vi "Feeding.vi"(8 "error In":errorcluster) -> (0 "error out":errorcluster)   [LabVIEW 2017]
uses:
  <vilib>/Utility/error.llb/DialogType.ctl
  Controls/Feed_Cyc_Data.ctl
  Controls/QUEUE_STATES.ctl
  Controls/Feed_St.ctl
  <vilib>/Utility/file.llb/Read Delimited Spreadsheet (string).vi
  Global/PLC_to_Auto.vi
  <vilib>/Instr/_visa.llb/VISA Configure Serial Port (Instr).vi
panel:
  in  "Door Number 2":i32
  out "Door Number":i32
  out "Door":bool
  out "number":i32
  out "Scanned Chld Part.Selected Door No":string
  out "output cluster":cluster{"Feeder Door Open":bool, "Address":u16}
  out "Scanned Chld Part":T1
  in  "Close _Door":bool
  out "raw scan code":string
  in  "Boolean":bool
  in  "String":string
  out "Bins/Box":i32
  out "Scanner Comm":bool
  out "Stop scanner":bool
  out "CYCLE STATUS":string
  out "CURRENT PLAN":T2
  out "SCAN CODE:":string
  out "Selected Plan structure":string[][](table)
  out "Plan Selected:":string
  out "USER:-":string
  in  "Stop":bool
  out "DATE/TIME":string
  out "Screen Name":string
  # "DOOR NUMBER"
  # "FEEDER STATUS"
  # "DOOR NUMBER"
  # "FEEDER STATUS"
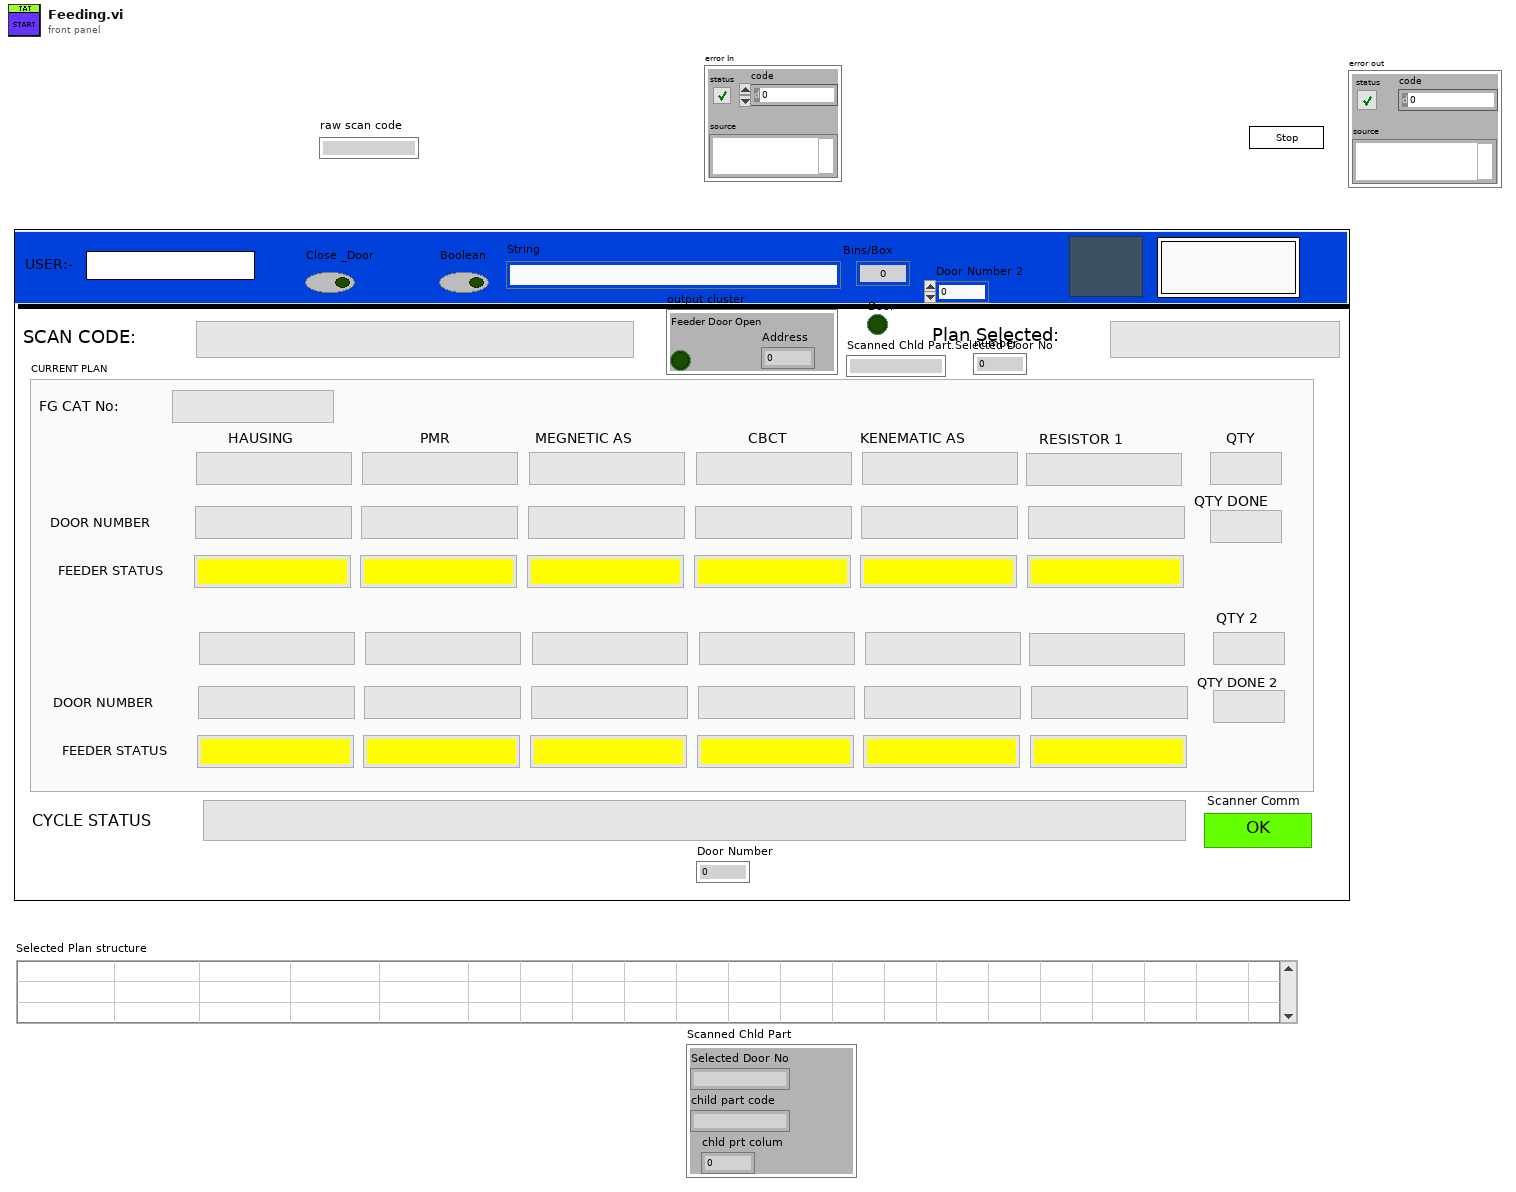
[diagram p1: front panel]
types:
  T1 = cluster{"Selected Door No":string, "child part code":string, "chld prt colum":i32}
  T2 = cluster{"FG CAT No:":string, "HAUSING":string, "PMR":string, "MEGNETIC AS":string, "CBCT":string, "KENEMATIC AS":string, "RESISTOR 1":string, "HAUSING DOOR":string, "PMR DOOR":string, "MAGNETIC AS DOOR":string, "CBCT DOOR":string, "KINEMATIC AS DOOR":string, "RESISTOR 1 DOOR":string, "HAUSING FEED STATUS":string, "PMR FEED STATUS":string, "MAGNETIC AS FEEED STATUS":string, "CBCT FEED STATUS":string, "KINEMATIC AS FEED STATUS":string, "RESISTOR 1 FEED STATUS":string, "QTY":string, "QTY DONE":string, "HAUSING 2":string, "PMR 2":string, "MEGNETIC AS 2":string, "CBCT 2":string, "KENEMATIC AS 2":string, "RESISTOR 2":string, "HAUSING DOOR 2":string, "PMR DOOR 2":string, "MAGNETIC AS DOOR 2":string, "CBCT DOOR 2":string, "KINEMATIC AS DOOR 2":string, "RESISTOR 1 DOOR 2":string, "HAUSING FEED STATUS 2":string, "PMR FEED STATUS 2":string, "MAGNETIC AS FEEED STATUS 2":string, "CBCT FEED STATUS 2":string, "KINEMATIC AS FEED STATUS 2":string, "RESISTOR 1 FEED STATUS 2":string, "QTY 2":string, "QTY DONE 2":string}
  T3 = typedef "Feed_Cyc_Data.ctl" = cluster{"Cycle_Plan":path, "Plan_Data":string[][], "Scanned_Data":string[], "Scanned Chld Part":cluster{"Selected Door No":string, "child part code":string, "chld prt Row":i32, "Chld Prt Index":i32, "Scanned Data":string}, "feed Status Indi":refnum<vi>[], "Recipe Selected":cluster{"Bin/Box Mode":i32, "Selected Section":i32}}
  T4 = typedef "DialogType.ctl" = u16
  T5 = enum32{"invalid app kind", "Development System", "Run Time System", "Student Edition", "Embedded LabVIEW", "Evaluation", "Custom"}
  T6 = typedef "QUEUE_STATES.ctl" = enum16{"CREATE Q", "EN Q", "DE Q", "CLOSE Q"}
  T7 = cluster{"Printer IP":string, "PLC IP Address":string, "Scanner Com":refnum<visa-resource-name>}
  T8 = typedef "Feed_St.ctl" = enum16{"Package_Qty_Count", "GENERATE_QR_PRNT", "Cluster_update", "Read_Plan", "QR_Scanned", "Int", "SaveReport ", "Open_Door", "Error_Handler", "Wait", "Close_Door", "Stop"}
  T9 = cluster{"Selected Door No":string, "child part code":string, "chld prt Row":i32, "Chld Prt Index":i32, "Scanned Data":string}
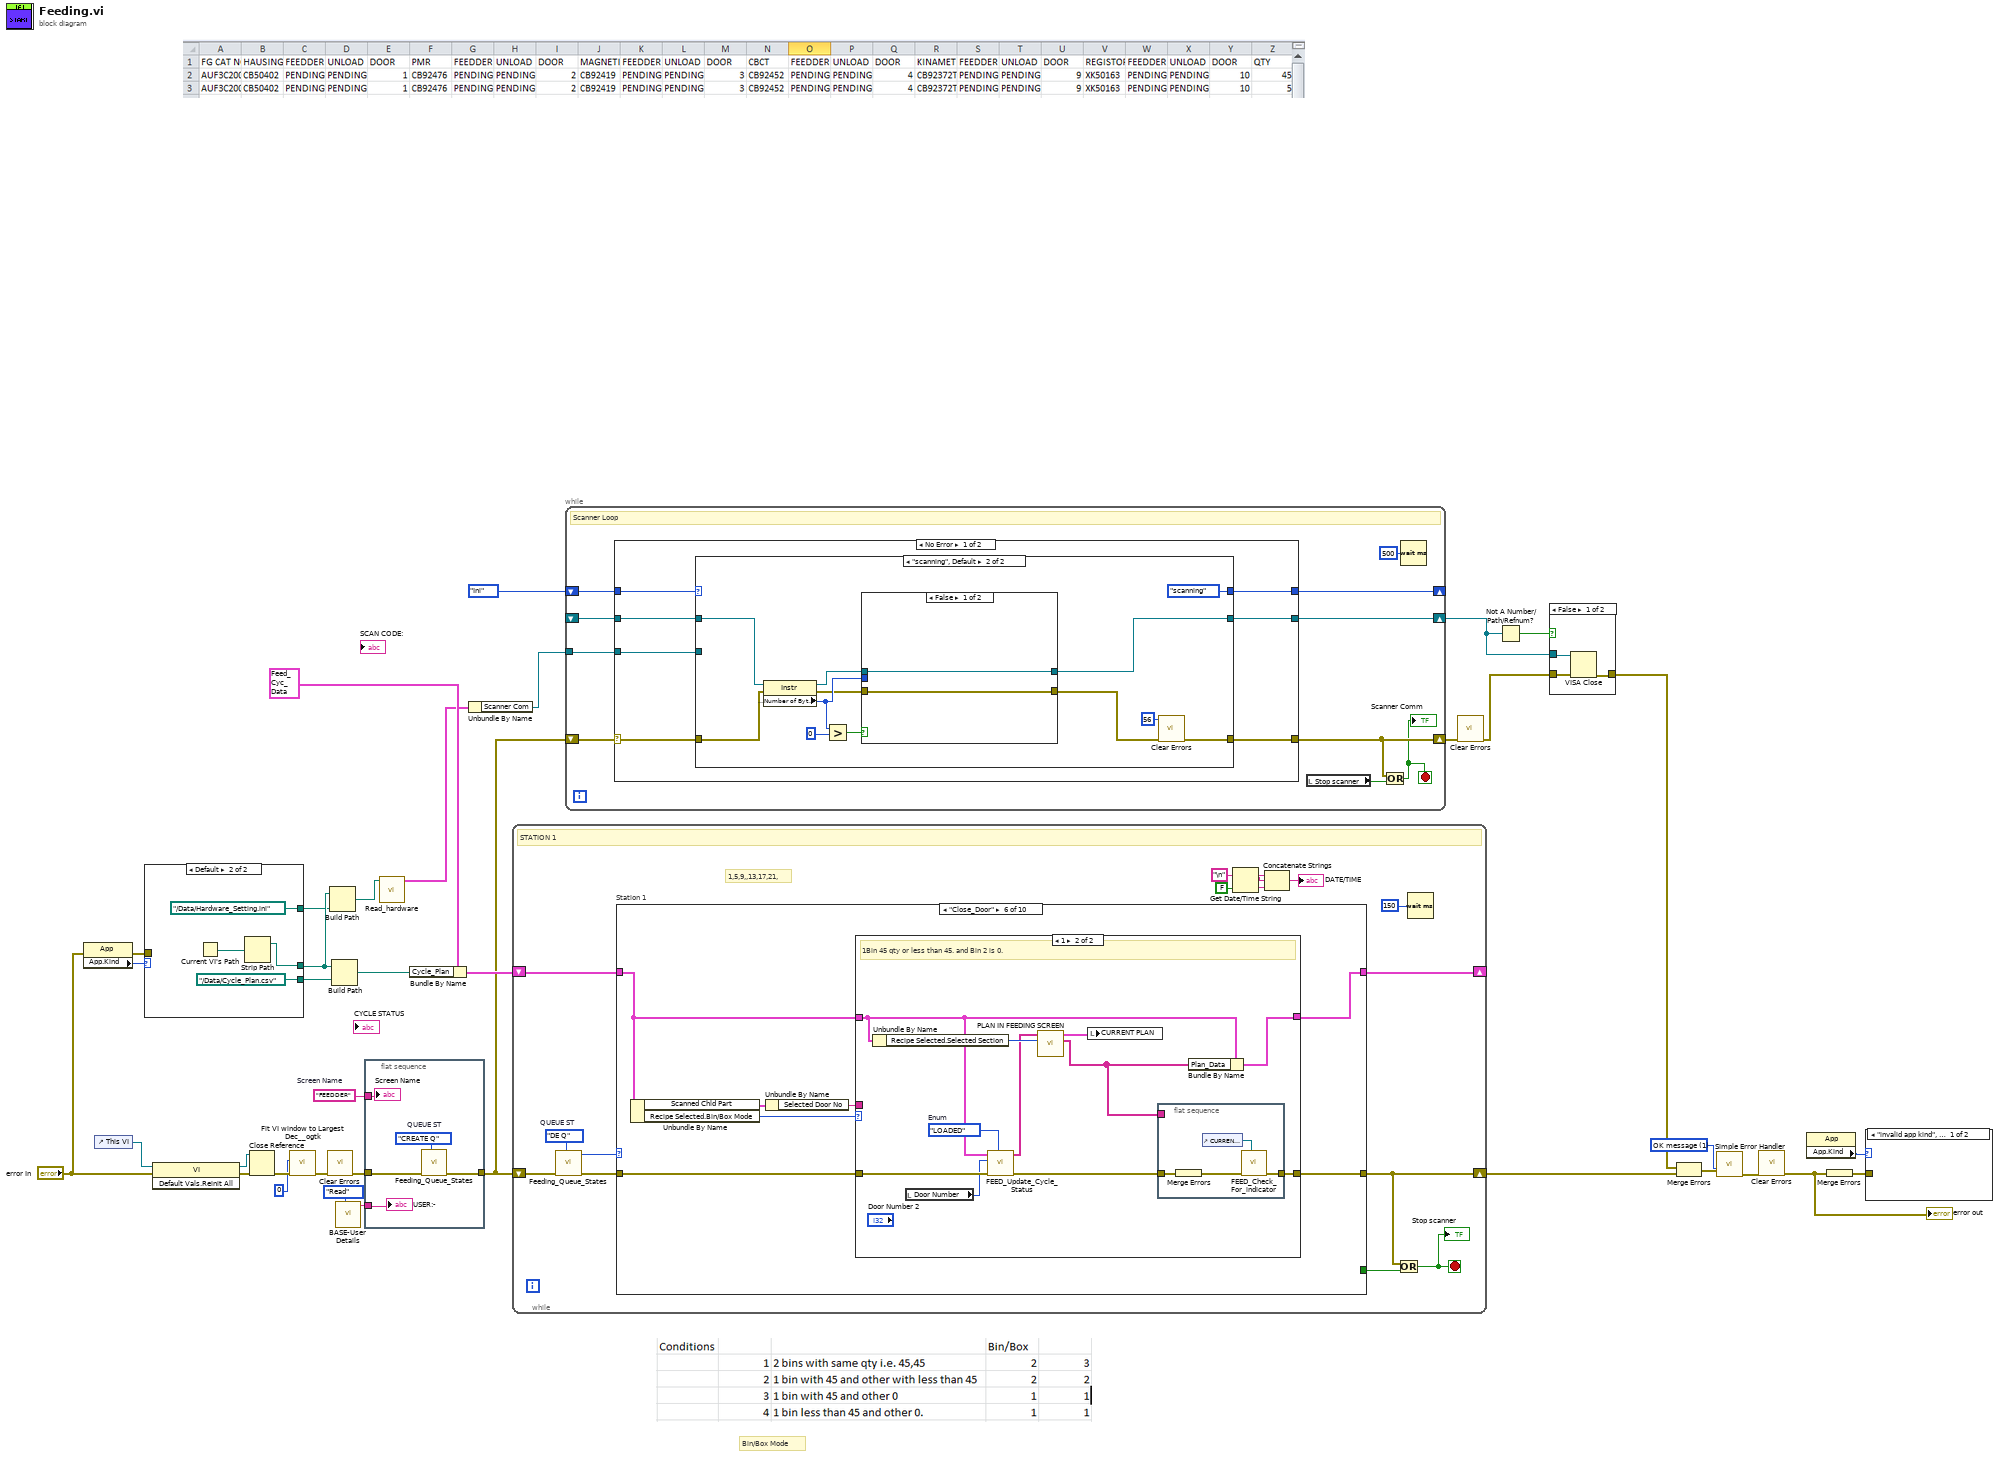
[diagram p0: block diagram]
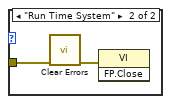
[diagram p2: hidden frame]
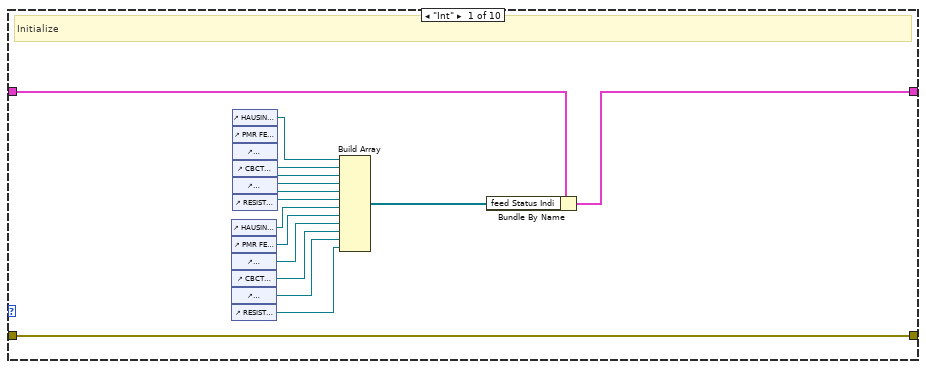
[diagram p3: hidden frame]
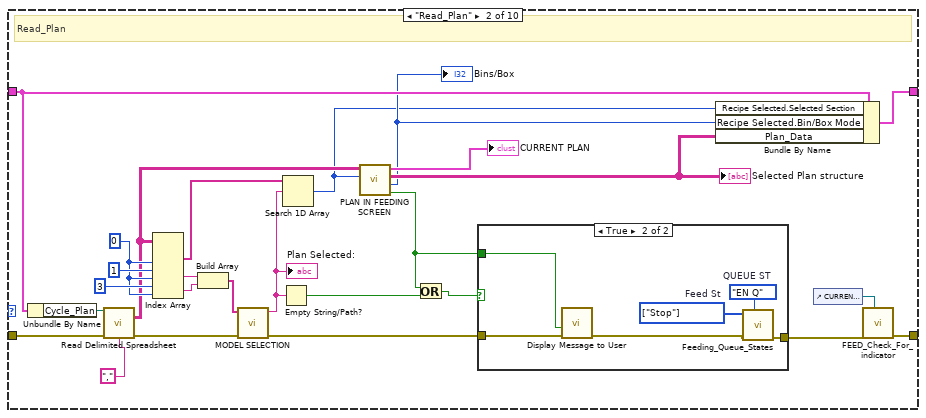
[diagram p4: hidden frame]
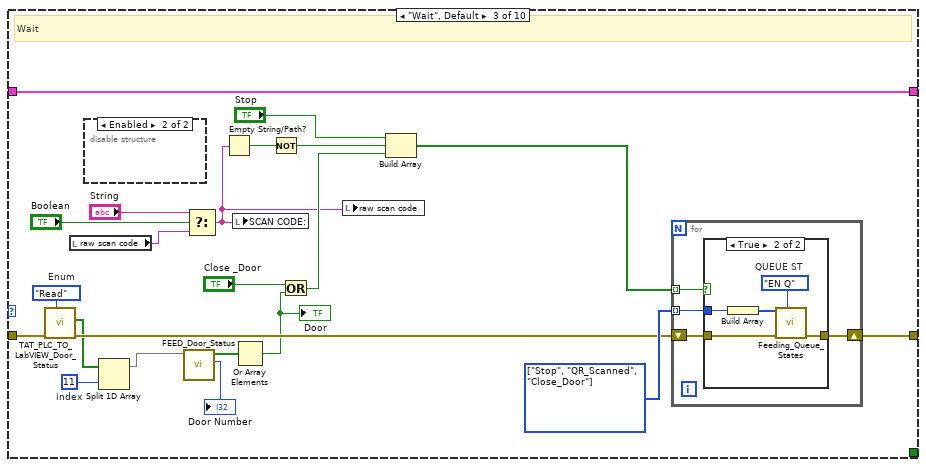
[diagram p6: hidden frame]
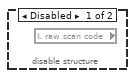
[diagram p7: hidden frame]
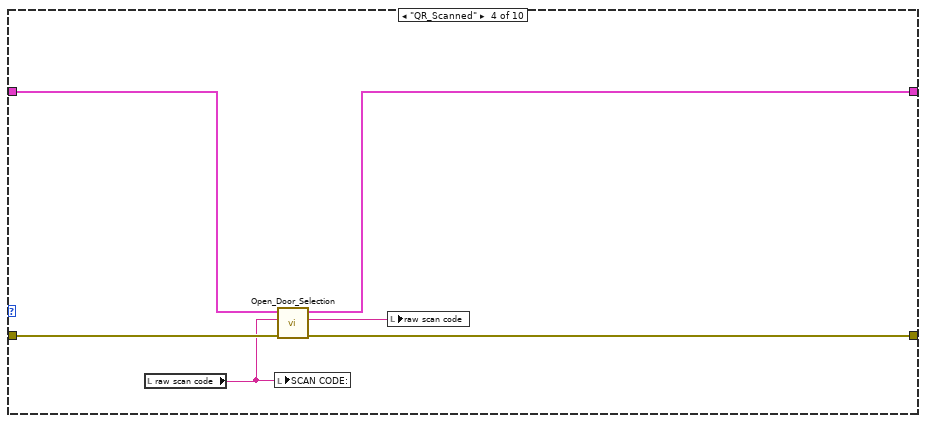
[diagram p9: hidden frame]
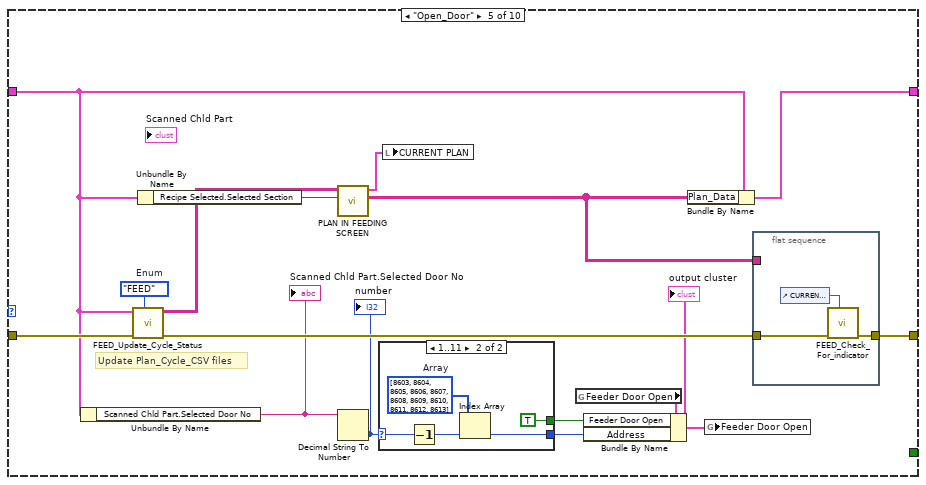
[diagram p10: hidden frame]
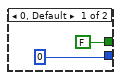
[diagram p11: hidden frame]
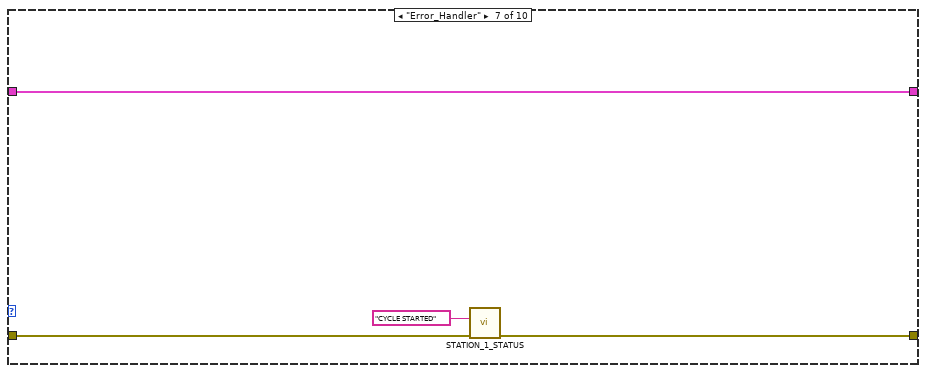
[diagram p13: hidden frame]
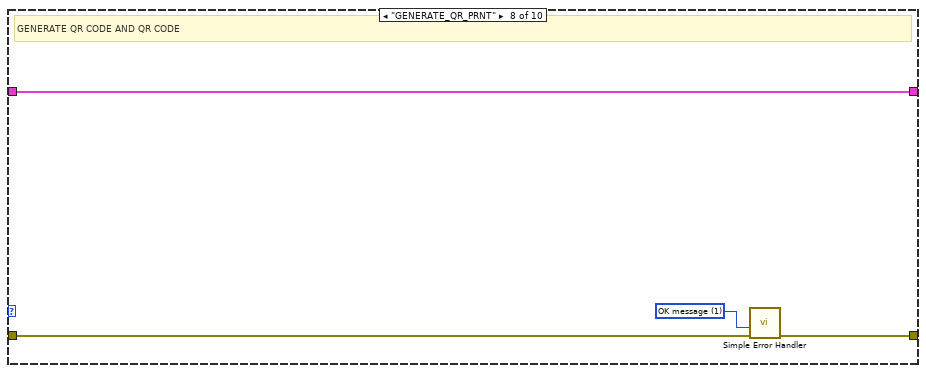
[diagram p14: hidden frame]
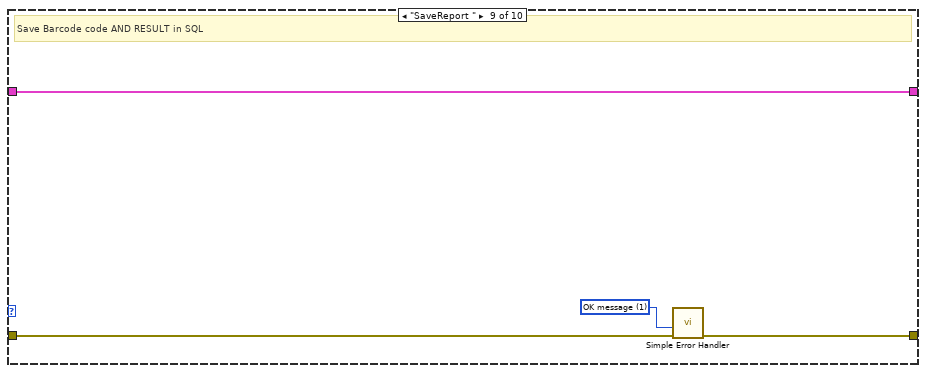
[diagram p15: hidden frame]
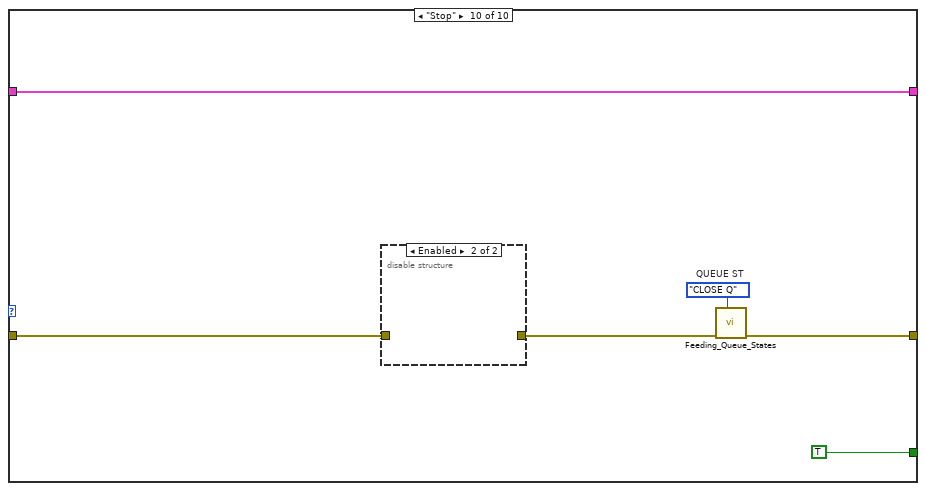
[diagram p16: hidden frame]
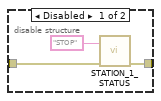
[diagram p17: hidden frame]
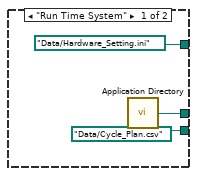
[diagram p18: hidden frame]
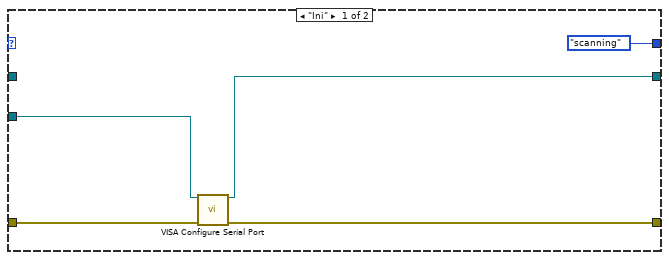
[diagram p20: hidden frame]
diagram:
  w17 = "FEEDDER"  # Screen Name
  w29 = T4 1 items=["no dialog", "OK message", "continue or stop message", "OK message + warnings", "continue/stop + warnings"] ("type of dialog (OK msg:1)")
  # "Bin/Box Mode"
  n1 = property class="App"(error in="error In") -> (error out=w25:errorcluster, "App.Kind"=w27:T5)  [unwired: 1 in, 1 out]
  n2 = control-ref of="This VI"() -> (w36:refnum<vi>)
  n3 = case shown="Default" w27 {
    tunnel: [path "Data/Cycle_Plan.csv" ("path") path "../Data/Cycle_Plan.csv" ("path")] -> w26
    tunnel: [w37 w41] -> w6
    tunnel: w25 -> [_ _]
    tunnel: [path "Data/Hardware_Setting.ini" ("path") path "../Data/Hardware_Setting.ini" ("path")] -> w5
    frame "Run Time System" {
      n4 = call <vilib>:"Application Directory.vi"() -> ("Application Directory"=w37:path)
    }
    frame Default {
      n5 = Current VI's Path() -> (path=w42:path)
      n6 = Strip Path(path=w42) -> (stripped path=w41:path)  [unwired: 1 out]
    }
  }
  n7 = invoke class="VI" method="Default Vals.Reinit All"(reference=w36, error in="error In") -> (reference out=w34:refnum<vi>, error out=w35:errorcluster)  [unwired: 1 in, 1 out]
  n8 = Close Reference(reference=w34, error in (no error)=w35) -> (error out=w33:errorcluster)
  n9 = call <userlib>:"Fit VI window to Largest Dec__ogtk.vi"("error in (no error)"=w33, "border spacing (2 px)"=0) -> ("error out"=w23:errorcluster)  [unwired: 4 in, 1 out]
  n10 = call <vilib>:"Clear Errors.vi"("error in (no error)"=w23) -> ("error out"=w10:errorcluster)  [unwired: 5 in, 1 out]
  n11 = Build Path(base path=w6, name or relative path=w5) -> (appended path=w4:path)
  n12 = Build Path(base path=w6, name or relative path=w26) -> (appended path=w19:path)
  n13 = call "BASE-User Details.vi"("Enum"=enum16{"Read", "Write"}."Read") -> ("User Name Out"=w30:string)  [unwired: 9 in, 1 out]
  n14 = flat-sequence {
    tunnel: [w45] -> w11
    tunnel: w10 -> [w46]
    tunnel: w30 -> [w48]
    tunnel: w17 -> [w47]
    frame #0 {
      w44 = QUEUE_STATES."CREATE Q"  # QUEUE ST
      n15 = call "Feeding_Queue_States.vi"("QUEUE ST"=w44, "error in"=w46) -> ("error OUT"=w45:errorcluster)  [unwired: 8 in, 1 out]
      "USER:-" <- w48
      "Screen Name" <- w47
    }
  }
  n16 = call "Read_hardware.vi"("configuration file path"=w4) -> ("data"=w8:T7)  [unwired: 10 in]
  n17 = Bundle By Name(cluster=T3 {"Cycle_Plan"=path "", "Plan_Data"=[], "Scanned_Data"=[], "Scanned Chld Part"={"Selected Door No"="", "child part code"="", "chld prt Row"=0, "Chld Prt Index"=0, "Scanned Data"=""}, "feed Status Indi"=[], "Recipe Selected"={"Bin/Box Mode"=0, "Selected Section"=0}}, "Cycle_Plan"=w19) -> (w18:T3)
  n18 = Unbundle By Name(w8) -> ("Scanner Com"=w7:refnum<visa-resource-name>)
  n19 = while {
    shift-right: [w55] -> _
    shift-left: w18 -> [w56]
    shift-right: [w53] -> w9
    shift-left: w11 -> [w52]
    stop <- w54 stop-if-true
    w50 = QUEUE_STATES."DE Q"  # QUEUE ST
    # "1,5,9,,13,17,21,"
    # "STATION 1"
    n20 = call "Feeding_Queue_States.vi"("QUEUE ST"=w50, "error in"=w52) -> ("error OUT"=w51:errorcluster, "Feed ST"=w49:T8)  [unwired: 8 in]
    n21 = case "Station 1" shown="\"Close_Door\"" w49 {
      tunnel: [_ _ _ _ _ _ _ _ _ TRUE] -> w57
      tunnel: [w79 w85 w131 w149 w164 w182 w202 w207 w211 w213] -> w53
      tunnel: w51 -> [w79 w104 w121 w150 w166 w183 w203 w206 w210 w217]
      tunnel: w56 -> [w66 w94 w134 w147 w157 w179 w201 w205 w209 w216]
      tunnel: [w65 w84 w134 w146 w161 w178 w201 w205 w209 w216] -> w55
      frame "Int" {
        # "Initialize"
        n22 = control-ref of="HAUSING FEED STATUS 2"() -> (w73:refnum<vi>)
        n23 = control-ref of="PMR FEED STATUS 2"() -> (w74:refnum<vi>)
        n24 = control-ref of="MAGNETIC AS FEEED STATUS 2"() -> (w75:refnum<vi>)
        n25 = control-ref of="CBCT FEED STATUS 2"() -> (w76:refnum<vi>)
        n26 = control-ref of="KINEMATIC AS FEED STATUS 2"() -> (w77:refnum<vi>)
        n27 = control-ref of="RESISTOR 1 FEED STATUS 2"() -> (w78:refnum<vi>)
        n28 = control-ref of="HAUSING FEED STATUS"() -> (w67:refnum<vi>)
        n29 = control-ref of="PMR FEED STATUS"() -> (w68:refnum<vi>)
        n30 = control-ref of="MAGNETIC AS FEEED STATUS"() -> (w69:refnum<vi>)
        n31 = control-ref of="CBCT FEED STATUS"() -> (w70:refnum<vi>)
        n32 = control-ref of="KINEMATIC AS FEED STATUS"() -> (w71:refnum<vi>)
        n33 = control-ref of="RESISTOR 1 FEED STATUS"() -> (w72:refnum<vi>)
        n34 = Build Array(w67, w68, w69, w70, w71, w72, w73, w74, w75, w76, w77, w78) -> (w64:refnum<vi>[])
        n35 = Bundle By Name(cluster=w66, "feed Status Indi"=w64) -> (w65:T3)
      }
      frame "Read_Plan" {
        w96 = 0
        # "Read_Plan"
        n36 = Unbundle By Name(w94) -> ("Cycle_Plan"=w103:path)
        n37 = call-poly <vilib>:"Read Delimited Spreadsheet.vi"("file path (dialog if empty)"=w103, "error in (no error)"=w104, "delimiter (\\t)"=",") -> ("all rows"=w90:string[][], "error out"=w97:errorcluster)  [unwired: 7 in, 4 out]
        n38 = Index Array(array=w90, index (col) #1=w96, index (row) #2=1, index (col) #2=w96, index (row) #3=3, index (col) #3=w96) -> (element #1=w95:string[], element #2=w100:string, element #3=w99:string)  [unwired: 1 in]
        n39 = Build Array(w100, w99) -> (w98:string[])
        n40 = call "MODEL SELECTION.vi"("error in (no error)"=w97, "Plan List"=w98) -> ("error out 2"=w88:errorcluster, "Plan Selected"=w93:string)  [unwired: 8 in]
        "Plan Selected:" <- w93
        n41 = Empty String/Path?(string/path=w93) -> (empty?=w87:bool)
        n42 = Search 1D Array(1D array=w95, element=w93) -> (index of element=w82:i32)  [unwired: 1 in]
        n43 = call "PLAN IN FEEDING SCREEN.vi"("Section selected"=w82, "PLAN In"=w90) -> ("FEED CMPLT?"=w80:bool, "Bin/Box"=w89:i32, "PLAN Out"=w91:string[][], "CURRENT PLAN"=→"CURRENT PLAN":T2)  [unwired: 6 in]
        "Selected Plan structure" <- w91
        "Bins/Box" <- w89
        n44 = Or(x=w80, y=w87) -> (x .or. y?=w81:bool)
        n45 = case shown="True" w81 {
          tunnel: w88 -> [w106 w109]
          tunnel: [w106 w111] -> w86
          tunnel: w80 -> [_ w107]
          frame False {
          }
          frame True {
            w110 = T8[] [enum."Stop"] items=["Package_Qty_Count", "GENERATE_QR_PRNT", "Cluster_update", "Read_Plan", "QR_Scanned", "Int", "SaveReport ", "Open_Door", "Error_Handler", "Wait", "Close_Door", "Stop"]  # Feed St
            w112 = QUEUE_STATES."EN Q"  # QUEUE ST
            n46 = call "Display Message to User"("error in (no error)"=w109, "Enable"=w107) -> ("error out"=w108:errorcluster)  [unwired: 8 in, 1 out]
            n47 = call "Feeding_Queue_States.vi"("QUEUE ST"=w112, "error in"=w108, "Feed St"=w110) -> ("error OUT"=w111:errorcluster)  [unwired: 7 in, 1 out]
          }
        }
        n48 = Bundle By Name(cluster=w94, "Recipe Selected.Selected Section"=w82, "Recipe Selected.Bin/Box Mode"=w89, "Plan_Data"=w91) -> (w84:T3)
        n49 = control-ref of="CURRENT PLAN"() -> (w83:refnum<vi>)
        n50 = call "FEED_Check_For_indicator.vi"("CURRENT PLAN"=w83, "error in (no error)"=w86) -> ("error out"=w85:errorcluster)  [unwired: 9 in]
      }
      frame "Wait", Default {
        w113 = 11  # index
        w124 = enum16{"Read", "Write"}."Read"  # Enum
        w127 = T8[] [enum."Stop", enum."QR_Scanned", enum."Close_Door"] items=["Package_Qty_Count", "GENERATE_QR_PRNT", "Cluster_update", "Read_Plan", "QR_Scanned", "Int", "SaveReport ", "Open_Door", "Error_Handler", "Wait", "Close_Door", "Stop"] ("Array")
        # "Wait"
        n51 = call "TAT_PLC_TO_LabVIEW_Door_Status.vi"("Enum"=w124, "error in (no error)"=w121) -> ("error out"=w120:errorcluster, "Array 2"=w115:bool[])  [unwired: 8 in]
        n52 = local read "raw scan code"() -> (w125:string)
        n53 = disable-structure shown="Enabled" {
          frame Disabled {
            n54 = local read "raw scan code"() -> ()  [unwired: 1 out]
          }
          frame Enabled {
          }
        }
        n55 = Split 1D Array(array=w115, index=w113) -> (first subarray=w114:bool[])  [unwired: 1 out]
        n56 = call "FEED_Door_Status.vi"("Array in"=w114) -> ("Door Number"=→"Door Number":i32, "Array out"=w119:bool[])  [unwired: 9 in]
        n57 = Select(t="String", s="Boolean", f=w125) -> (s? t:f=w116:string)
        n58 = Empty String/Path?(string/path=w116) -> (empty?=w130:bool)
        n59 = local write "SCAN CODE:"(w116) -> ()
        n60 = Or Array Elements(Boolean array=w119) -> (logical OR=w118:bool)
        "Door" <- w118
        n61 = Not(x=w130) -> (.not. x?=w126:bool)
        n62 = Or(x="Close _Door", y=w118) -> (x .or. y?=w122:bool)
        n63 = local write "raw scan code"(w116) -> ()
        n64 = Build Array("Stop", w126, w122) -> (w128:bool[])
        n65 = for {
          shift-right: [w137] -> w131
          shift-left: w120 -> [w138]
          tunnel: w128 -> [w136] mode=indexing
          tunnel: w127 -> [w135] mode=indexing
          n66 = case shown="True" w136 {
            tunnel: w138 -> [w139 w143]
            tunnel: [w139 w142] -> w137
            tunnel: w135 -> [_ w141]
            frame False {
            }
            frame True {
              w144 = QUEUE_STATES."EN Q"  # QUEUE ST
              n67 = Build Array(w141) -> (w140:T8[])
              n68 = call "Feeding_Queue_States.vi"("QUEUE ST"=w144, "error in"=w143, "Feed St"=w140) -> ("error OUT"=w142:errorcluster)  [unwired: 7 in, 1 out]
            }
          }
        }
      }
      frame "QR_Scanned" {
        n69 = local read "raw scan code"() -> (w148:string)
        n70 = local write "SCAN CODE:"(w148) -> ()
        n71 = call "Open_Door_Selection.vi"("error in (no error)"=w150, "raw scan code"=w148, "Cluster In"=w147) -> ("error out"=w149:errorcluster, "String"=w145:string, "Cluster Out"=w146:T3)  [unwired: 6 in]
        n72 = local write "raw scan code"(w145) -> ()
      }
      frame "Open_Door" {
        w159 = enum16{"FEED", "LOADED"}."FEED"  # Enum
        # "Update Plan_Cycle_CSV files"
        n73 = Unbundle By Name(w157) -> ("Scanned Chld Part.Selected Door No"=w153:string)
        "Scanned Chld Part.Selected Door No" <- w153
        n74 = call "FEED_Update_Cycle_Status.vi"("Enum"=w159, "error in (no error)"=w166, 11:w157) -> ("error out"=w165:errorcluster, "output array"=w158:string[][])  [unwired: 6 in, 1 out]
        n75 = Unbundle By Name(w157) -> ("Recipe Selected.Selected Section"=w163:i32)
        n76 = call "PLAN IN FEEDING SCREEN.vi"("Section selected"=w163, "PLAN In"=w158) -> ("PLAN Out"=w160:string[][], "CURRENT PLAN"=w162:T2)  [unwired: 6 in, 2 out]
        n77 = Decimal String To Number(string=w153) -> (number=w154:i32)  [unwired: 2 in, 1 out]
        "number" <- w154
        n78 = case shown="1..11" w154 {
          selector: w154 -> [_ w173]
          tunnel: [u16 0 w172] -> w152
          tunnel: [FALSE TRUE] -> w151
          frame 0, Default {
          }
          frame 1..11 {
            w169 = i32[] [8603, 8604, 8605, 8606, 8607, 8608, 8609, 8610, 8611, 8612, 8613]  # Array
            n79 = Decrement(x=w173) -> (x-1=w170:i32)
            n80 = Index Array(array=w169, index=w170) -> (element=w172:i32)
          }
        }
        n81 = local write "CURRENT PLAN"(w162) -> ()
        n82 = global read "PLC_to_Auto.vi" "Feeder Door Open"() -> (w156:cluster{"Feeder Door Open":bool, "Address":u16})
        n83 = Bundle By Name(cluster=w156, "Feeder Door Open"=w151, "Address"=w152) -> (w155:cluster{"Feeder Door Open":bool, "Address":u16})
        "output cluster" <- w155
        n84 = Bundle By Name(cluster=w157, "Plan_Data"=w160) -> (w161:T3)
        n85 = global write "PLC_to_Auto.vi" "Feeder Door Open"(w155) -> ()
        n86 = flat-sequence {
          tunnel: w165 -> [w176]
          tunnel: [w175] -> w164
          tunnel: w160 -> [_]
          frame #0 {
            n87 = control-ref of="CURRENT PLAN"() -> (w174:refnum<vi>)
            n88 = call "FEED_Check_For_indicator.vi"("CURRENT PLAN"=w174, "error in (no error)"=w176) -> ("error out"=w175:errorcluster)  [unwired: 9 in]
          }
        }
      }
      frame "Close_Door" {
        n89 = Unbundle By Name(w179) -> ("Scanned Chld Part"=w180:T9, "Recipe Selected.Bin/Box Mode"=w177:i32)
        n90 = Unbundle By Name(w180) -> ("Selected Door No"=w181:string)
        n91 = case shown="1" w177 {
          tunnel: w183 -> [w184 w195]
          tunnel: [w184 w188] -> w182
          tunnel: w181 -> [_ _]
          tunnel: w179 -> [w185 w190]
          tunnel: [w185 w196] -> w178
          frame 0, Default {
          }
          frame 1 {
            w193 = enum16{"FEED", "LOADED"}."LOADED"  # Enum
            # "1Bin 45 qty or less than 45. and Bin 2 is 0."
            n92 = Unbundle By Name(w190) -> ("Recipe Selected.Selected Section"=w192:i32)
            n93 = local read "Door Number"() -> (w186:i32)
            n94 = call "FEED_Update_Cycle_Status.vi"("Enum"=w193, "error in (no error)"=w195, "Door No"=w186, 11:w190) -> ("error out"=w194:errorcluster, "output array"=w189:string[][])  [unwired: 5 in, 1 out]
            n95 = call "PLAN IN FEEDING SCREEN.vi"("Section selected"=w192, "PLAN In"=w189) -> ("PLAN Out"=w187:string[][], "CURRENT PLAN"=w191:T2)  [unwired: 6 in, 2 out]
            n96 = local write "CURRENT PLAN"(w191) -> ()
            n97 = flat-sequence {
              tunnel: w194 -> [w200]
              tunnel: [w197] -> w188
              tunnel: w187 -> [_]
              frame #0 {
                n98 = Merge Errors(w200) -> (w198:errorcluster)
                n99 = control-ref of="CURRENT PLAN"() -> (w199:refnum<vi>)
                n100 = call "FEED_Check_For_indicator.vi"("CURRENT PLAN"=w199, "error in (no error)"=w198) -> ("error out"=w197:errorcluster)  [unwired: 9 in]
              }
            }
            n101 = Bundle By Name(cluster=w190, "Plan_Data"=w187) -> (w196:T3)
          }
        }
      }
      frame "Error_Handler" {
        n102 = call "STATION_1_STATUS.vi"("error in (no error)"=w203, "STATUS"="CYCLE STARTED" ("Cycle Status")) -> ("error out"=w202:errorcluster)  [unwired: 9 in]
      }
      frame "GENERATE_QR_PRNT" {
        w208 = T4 1 items=["no dialog", "OK message", "continue or stop message", "OK message + warnings", "continue/stop + warnings"] ("type of dialog (OK msg:1)")
        # "GENERATE QR CODE AND QR CODE"
        n103 = call <vilib>:"Simple Error Handler.vi"("type of dialog (OK msg:1)"=w208, "error in (no error)"=w206) -> ("error out"=w207:errorcluster)  [unwired: 3 in, 4 out]
      }
      frame "SaveReport " {
        w212 = T4 1 items=["no dialog", "OK message", "continue or stop message", "OK message + warnings", "continue/stop + warnings"] ("type of dialog (OK msg:1)")
        # "Save Barcode code AND RESULT in SQL"
        n104 = call <vilib>:"Simple Error Handler.vi"("type of dialog (OK msg:1)"=w212, "error in (no error)"=w210) -> ("error out"=w211:errorcluster)  [unwired: 3 in, 4 out]
      }
      frame "Stop" {
        w215 = QUEUE_STATES."CLOSE Q"  # QUEUE ST
        n105 = disable-structure shown="Enabled" {
          disable-tunnel: w217 -> [w220 _]
          disable-tunnel: [w219 _] -> w214
          frame Disabled {
            n106 = call "STATION_1_STATUS.vi"("error in (no error)"=w220, "STATUS"="STOP" ("Cycle Status")) -> ("error out"=w219:errorcluster)  [unwired: 9 in]
          }
          frame Enabled {
          }
        }
        n107 = call "Feeding_Queue_States.vi"("QUEUE ST"=w215, "error in"=w214) -> ("error OUT"=w213:errorcluster)  [unwired: 8 in, 1 out]
      }
    }
    n108 = Get Date/Time String(want seconds? (F)=FALSE) -> (date string=w61:string, time string=w60:string)  [unwired: 2 in]
    n109 = Concatenate Strings(w61, "\n", w60) -> (→"DATE/TIME":string)
    n110 = Or(x=w53, y=w57) -> (x .or. y?=w54:bool)
    "Stop scanner" <- w54
    n111 = Wait (ms)(milliseconds to wait=u32 150) -> ()  [unwired: 1 out]
  }
  n112 = while {
    shift-right: [w230] -> w15
    shift-left: w11 -> [w231]
    shift-right: [w228] -> _
    shift-left: enum16{"Ini", "scanning", "Close"}."Ini" -> [w229]
    tunnel: w7 -> [w227]
    shift-right: [w226] -> w12
    shift-left: _ -> [w225]
    stop <- w224 stop-if-true
    # "Scanner Loop"
    n113 = case shown="No Error" w231 {
      selector: w231 -> [w238 w268]
      tunnel: [w237 w267] -> w230
      tunnel: w229 -> [w236 _]
      tunnel: [w235 enum16{"Ini", "scanning", "Close"}."scanning"] -> w228
      tunnel: w227 -> [w234 _]
      tunnel: [w233 w265] -> w226
      tunnel: w225 -> [w232 w265]
      frame No Error {
        n114 = case shown="\"scanning\", Default" w236 {
          tunnel: w238 -> [w242 w246]
          tunnel: [w241 w254] -> w237
          tunnel: [enum16{"Ini", "scanning", "Close"}."scanning" enum16{"Ini", "scanning", "Close"}."scanning"] -> w235
          tunnel: w234 -> [w240 _]
          tunnel: [w239 w244] -> w233
          tunnel: w232 -> [_ w247]
          frame "Ini" {
            n115 = call-poly "VISA Configure Serial Port"("VISA resource name"=w240, "error in (no error)"=w242) -> ("VISA resource name out"=w239:refnum<visa-resource-name>, "error out"=w241:errorcluster)  [unwired: 12 in]
          }
          frame "scanning", Default {
            n116 = property class="Instr"(reference=w247, error in=w246) -> (reference out=w249:refnum<visa-resource-name>, error out=w250:errorcluster, "Serial Settings:Number of Bytes at Serial Port"=w251:u32)
            n117 = Greater?(x=w251, y=u32 0) -> (0:w252:bool)
            n118 = case shown="False" w252 {
              tunnel: w249 -> [w257 w264]
              tunnel: w250 -> [w256 w263]
              tunnel: w251 -> [_ w262]
              tunnel: [w257 w261] -> w244
              tunnel: [w256 w259] -> w245
              frame False {
              }
              frame True {
                n119 = VISA Read(VISA resource name=w264, byte count=w262, error in (no error)=w263) -> (VISA resource name out=w261:refnum<visa-resource-name>, read buffer=w260:string, error out=w259:errorcluster)  [unwired: 1 out]
                n120 = call <vilib>:"Trim Whitespace.vi"("string"=w260) -> ("trimmed string"=→"raw scan code":string)  [unwired: 1 in]
              }
            }
            n121 = call <vilib>:"Clear Errors.vi"("error in (no error)"=w245, "specific error code to clear (0: all)"=56) -> ("error out"=w254:errorcluster)  [unwired: 4 in, 1 out]
          }
        }
      }
      frame Error {
        n122 = Unbundle By Name(w268) -> ("code"=w269:i32)
        n123 = case shown="1" w269 {
          tunnel: w268 -> [w273 w275]
          tunnel: [w271 w274] -> w267
          frame 0, Default {
            w270 = T4 2 items=["no dialog", "OK message", "continue or stop message", "OK message + warnings", "continue/stop + warnings"] ("type of dialog (OK msg:1)")
            n124 = call <vilib>:"Simple Error Handler.vi"("type of dialog (OK msg:1)"=w270, "error in (no error)"=w273) -> ("error out"=w272:errorcluster)  [unwired: 3 in, 4 out]
            n125 = call <vilib>:"Clear Errors.vi"("error in (no error)"=w272) -> ("error out"=w271:errorcluster)  [unwired: 5 in, 1 out]
          }
          frame 1 {
            w276 = "THIS ERROR OCCURED AS SCREEN 1 IS NOT CONNECTED OR OFF"  # source
            # "Monitor not present/Off/disconnected"
            n126 = Bundle By Name(cluster=w275, "source"=w276) -> (w274:errorcluster)
          }
        }
      }
    }
    n127 = local read "Stop scanner"() -> (w222:bool)
    n128 = Or(x=w230, y=w222) -> (x .or. y?=w224:bool)
    "Scanner Comm" <- w224
    n129 = Wait (ms)(milliseconds to wait=u32 500) -> ()  [unwired: 1 out]
  }
  n130 = call <vilib>:"Clear Errors.vi"("error in (no error)"=w15) -> ("error out"=w13:errorcluster)  [unwired: 5 in, 1 out]
  n131 = Not A Number/Path/Refnum?(number/path/refnum=w12) -> (NaN/Path/Refnum?=w14:bool)
  n132 = case shown="False" w14 {
    tunnel: w13 -> [w279 w280]
    tunnel: w12 -> [w277 _]
    tunnel: [w278 w280] -> w3
    frame False {
      n133 = VISA Close(VISA resource name=w277, error in (no error)=w279) -> (error out=w278:errorcluster)
    }
    frame True {
    }
  }
  n134 = Merge Errors(w3, w9) -> (w32:errorcluster)
  n135 = call <vilib>:"Simple Error Handler.vi"("type of dialog (OK msg:1)"=w29, "error in (no error)"=w32) -> ("error out"=w2:errorcluster)  [unwired: 3 in, 4 out]
  n136 = call <vilib>:"Clear Errors.vi"("error in (no error)"=w2) -> ("error out"=w1:errorcluster)  [unwired: 5 in, 1 out]
  "error out" <- w1
  n137 = property class="App"() -> ("App.Kind"=w28:T5)  [unwired: 2 in, 2 out]
  n138 = Merge Errors(w1) -> (w21:errorcluster)
  n139 = case shown="\"invalid app kind\", Default" w28 {
    tunnel: w21 -> [_ w282]
    frame "invalid app kind", Default {
    }
    frame "Run Time System" {
      n140 = call <vilib>:"Clear Errors.vi"("error in (no error)"=w282) -> ("error out"=w281:errorcluster)  [unwired: 5 in, 1 out]
      n141 = invoke class="VI" method="FP.Close"(error in=w281) -> ()  [unwired: 2 in, 3 out]
    }
  }
